vi "Write Bias Voltage Index.vi"(10 "Bias Voltage Index":i32, 11 "LCR-Measurement in":refnum<class "LCR-Meas.lvclass">) -> (3 "LCR-Measurement out":refnum<class "LCR-Meas.lvclass">)   [LabVIEW 2020, in "LCR-Meas.lvclass"]
uses:
  LCR-Meas.lvclass
  LCR-Meas.lvclass/LCR-Meas.ctl
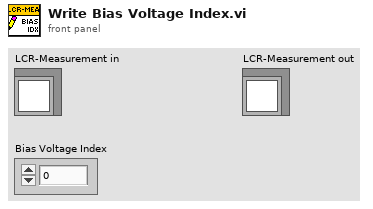
[diagram p1: front panel]
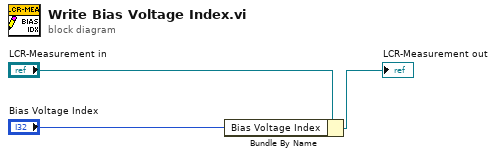
[diagram p0: block diagram]
diagram:
  n1 = Bundle By Name(cluster="LCR-Measurement in", "Bias Voltage Index"="Bias Voltage Index") -> (→"LCR-Measurement out":refnum<class "LCR-Meas.lvclass">)
